vi "HACH全局.vi"() -> ()   [LabVIEW 2016, in "HACH多参.lvlib"]
panel:
  in  "运行状态":string
  in  "显示值":T1
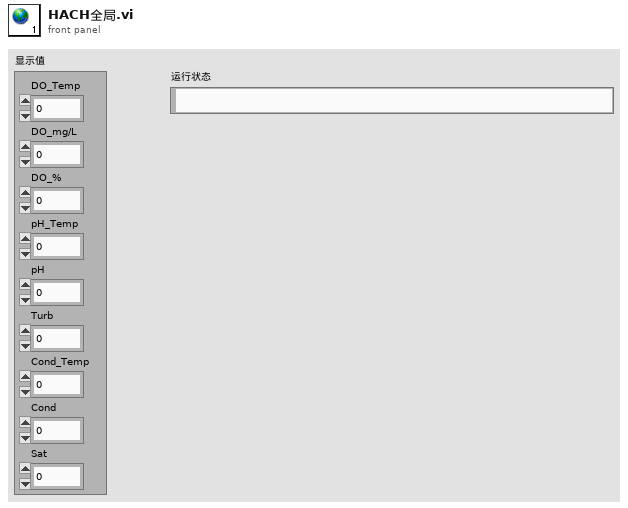
[diagram p1: front panel]
types:
  T1 = cluster{"DO_Temp":dbl, "DO_mg/L":dbl, "DO_%":dbl, "pH_Temp":dbl, "pH":dbl, "Turb":dbl, "Cond_Temp":dbl, "Cond":dbl, "Sat":dbl}
diagram:
